vi "Icon_2D Array Build Region.vi"(8 "Error":errorcluster, 11 "2D Image":T2) -> (0 "Error Out":errorcluster, 3 "Region Out":T3, 5 "Position Out":T1)   [LabVIEW 2009]
uses:
  Controls/Cluster/Cluster_Region info.ctl
  Controls/Cluster/Cluster_Top Left position.ctl
  Controls/Array/Color Box Array_2D Icon Viewer.ctl
  Controls/Enum/RBENUM_Icon Position.ctl
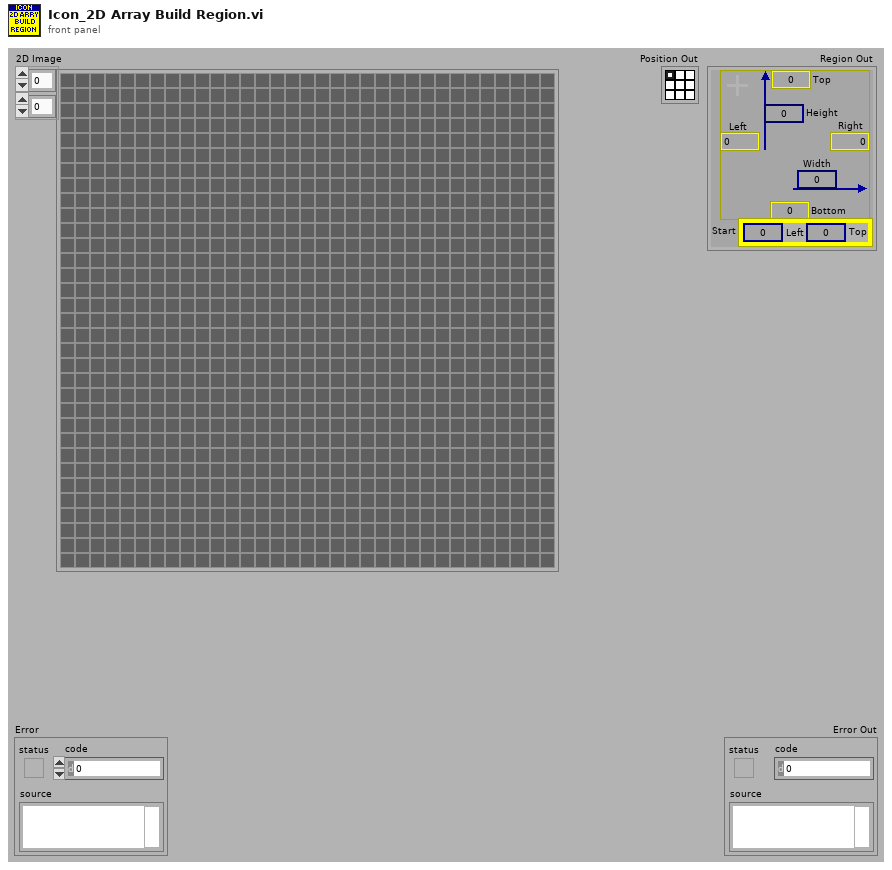
[diagram p1: front panel]
types:
  T1 = typedef "RBENUM_Icon Position.ctl" = enum32{"LFT-TOP", "MID-TOP", "RGT-TOP", "LFT-CTR", "MID-CTR", "RGT-CTR", "LFT-BOT", "MID-BOT", "RGT-BOT"}
  T2 = typedef "Color Box Array_2D Icon Viewer.ctl" = u32[][]
  T3 = typedef "Cluster_Region info.ctl" = cluster{"Left":i32, "Top":i32, "Right":i32, "Bottom":i32, "Width":u32, "Height":u32, "Start":T4}
  T4 = typedef "Cluster_Top Left position.ctl" = cluster{"Left":i32, "Top":i32}
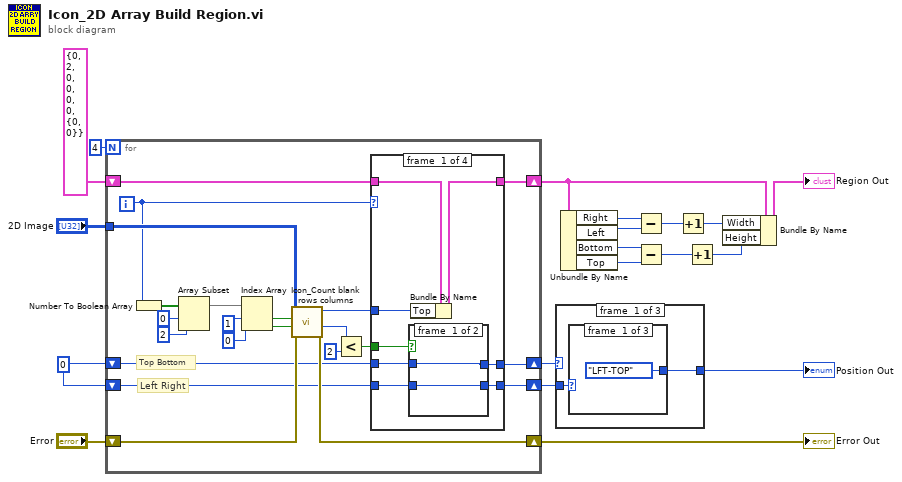
[diagram p0: block diagram]
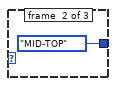
[diagram p2: hidden frame]
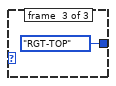
[diagram p3: hidden frame]
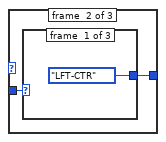
[diagram p4: hidden frame]
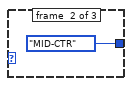
[diagram p5: hidden frame]
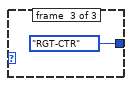
[diagram p6: hidden frame]
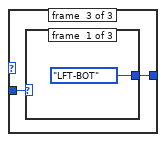
[diagram p7: hidden frame]
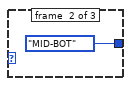
[diagram p8: hidden frame]
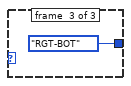
[diagram p9: hidden frame]
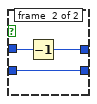
[diagram p10: hidden frame]
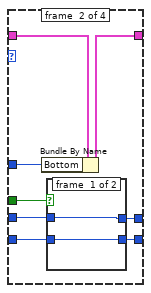
[diagram p11: hidden frame]
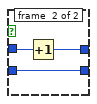
[diagram p12: hidden frame]
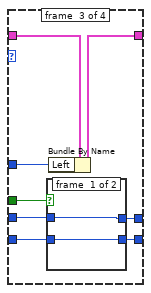
[diagram p13: hidden frame]
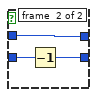
[diagram p14: hidden frame]
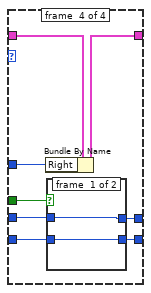
[diagram p15: hidden frame]
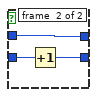
[diagram p16: hidden frame]
diagram:
  w4 = 0 ("Top")
  n1 = for {
    N: 4 -> [_]
    tunnel: "2D Image" -> [w39]
    shift-right: [w40] -> w11
    shift-left: "Error" -> [w41]
    shift-right: [w33] -> w18
    shift-left: T3 {"Left"=0, "Top"=2, "Right"=0, "Bottom"=0, "Width"=0, "Height"=0, "Start"={"Left"=0, "Top"=0}} ("Bounds Rect") -> [w34]
    shift-right: [w21] -> w3
    shift-left: w4 -> [w25]
    shift-right: [w20] -> w2
    shift-left: w4 -> [w24]
    i -> [w30]
    # "Top Bottom"
    # "Left Right"
    n2 = Number To Boolean Array(number=w30) -> (Boolean array=w28:bool[])
    n3 = Array Subset(array=w28, index=0, length=2) -> (w29:bool[])
    n4 = Index Array(array=w29, index #1=1 ("index"), index #2=0 ("index")) -> (element #1=w36:bool, element #2=w35:bool)
    n5 = call "Icon_Count blank rows columns.vi"("Error"=w41, "Near (f)\nfar (t)"=w35, "Height (f)\nWidth (t)"=w36, "2D Image"=w39) -> ("Error Out"=w40:errorcluster, "Blank Row count"=w31:i32, "Last Index Out"=w32:i32)  [unwired: 5 in]
    n6 = Less?(x=w31, y=2) -> (x < y?=w23:bool)
    n7 = case shown="3.." w30 {
      tunnel: w34 -> [w49 w62 w75 w88]
      tunnel: [w48 w61 w74 w87] -> w33
      tunnel: w32 -> [w47 w60 w73 w86]
      tunnel: w23 -> [w46 w59 w72 w85]
      tunnel: w25 -> [w45 w58 w71 w84]
      tunnel: w24 -> [w43 w56 w69 w82]
      tunnel: [w44 w57 w70 w83] -> w21
      tunnel: [w42 w55 w68 w81] -> w20
      frame #0 {
        n8 = case shown="False" w46 {
          tunnel: w45 -> [w51 w54]
          tunnel: [w51 w53] -> w44
          tunnel: w43 -> [w50 w52]
          tunnel: [w50 w52] -> w42
          frame #0 {
          }
          frame #1 {
            n9 = Decrement(x=w54) -> (x-1=w53:i32)
          }
        }
        n10 = Bundle By Name(cluster=w49, "Top"=w47) -> (w48:T3)
      }
      frame #1 {
        n11 = Bundle By Name(cluster=w62, "Bottom"=w60) -> (w61:T3)
        n12 = case shown="False" w59 {
          tunnel: w58 -> [w64 w67]
          tunnel: [w64 w66] -> w57
          tunnel: w56 -> [w63 w65]
          tunnel: [w63 w65] -> w55
          frame #0 {
          }
          frame #1 {
            n13 = Increment(x=w67) -> (x+1=w66:i32)
          }
        }
      }
      frame #2 {
        n14 = case shown="True" w72 {
          tunnel: w71 -> [w77 w79]
          tunnel: [w77 w79] -> w70
          tunnel: w69 -> [w76 w80]
          tunnel: [w76 w78] -> w68
          frame #0 {
          }
          frame #1 {
            n15 = Decrement(x=w80) -> (x-1=w78:i32)
          }
        }
        n16 = Bundle By Name(cluster=w75, "Left"=w73) -> (w74:T3)
      }
      frame #3 {
        n17 = Bundle By Name(cluster=w88, "Right"=w86) -> (w87:T3)
        n18 = case shown="True" w85 {
          tunnel: w84 -> [w90 w92]
          tunnel: [w90 w92] -> w83
          tunnel: w82 -> [w89 w93]
          tunnel: [w89 w91] -> w81
          frame #0 {
          }
          frame #1 {
            n19 = Increment(x=w93) -> (x+1=w91:i32)
          }
        }
      }
    }
  }
  "Error Out" <- w11
  n20 = case shown="0" w3 {
    tunnel: w2 -> [w95 w100 w105]
    tunnel: [w94 w99 w104] -> w1
    frame #0 {
      n21 = case shown="0" w95 {
        tunnel: [RBENUM_Icon_Position."LFT-TOP" ("Position") RBENUM_Icon_Position."MID-TOP" ("Position") RBENUM_Icon_Position."RGT-TOP" ("Position")] -> w94
        frame #0 {
        }
        frame #1 {
        }
        frame #2 {
        }
      }
    }
    frame #1 {
      n22 = case shown="0" w100 {
        tunnel: [RBENUM_Icon_Position."LFT-CTR" ("Position") RBENUM_Icon_Position."MID-CTR" ("Position") RBENUM_Icon_Position."RGT-CTR" ("Position")] -> w99
        frame #0 {
        }
        frame #1 {
        }
        frame #2 {
        }
      }
    }
    frame #2 {
      n23 = case shown="1.." w105 {
        tunnel: [RBENUM_Icon_Position."LFT-BOT" ("Position") RBENUM_Icon_Position."MID-BOT" ("Position") RBENUM_Icon_Position."RGT-BOT" ("Position")] -> w104
        frame #0 {
        }
        frame #1 {
        }
        frame #2 {
        }
      }
    }
  }
  "Position Out" <- w1
  n24 = Unbundle By Name(w18) -> ("Right"=w14:i32, "Left"=w15:i32, "Bottom"=w16:i32, "Top"=w17:i32)
  n25 = Subtract(x=w14, y=w15) -> (x-y=w9:i32)
  n26 = Subtract(x=w16, y=w17) -> (x-y=w8:i32)
  n27 = Increment(x=w9) -> (x+1=w7:i32)
  n28 = Increment(x=w8) -> (x+1=w6:i32)
  n29 = Bundle By Name(cluster=w18, "Width"=w7, "Height"=w6) -> (→"Region Out":T3)
